vi "Best Focus.vi"(7 "Use Strength?":bool, 8 "error in (no error)":errorcluster, 9 "Inc by":dbl=-0.1 format="%#_13g", 10 "Start":dbl=1.0 format="%#_13g", 11 "Gantry In":refnum<k24>) -> (0 "error out":errorcluster, 2 "max value":dbl, 3 "Gantry Out":refnum<k24>)   [LabVIEW 2021, in "Component Tray.lvclass"]
uses:
  Component Tray.lvclass
  C:/Program Files (x86)/Aerotech/A3200/LabVIEW/2010/Bin/Aerotech.A3200.dll
  Program Files (x86)/Aerotech/A3200/LabVIEW/2010/Bin/Aerotech.A3200.dll
  Controller/Motion/A3200/A3200.lvclass
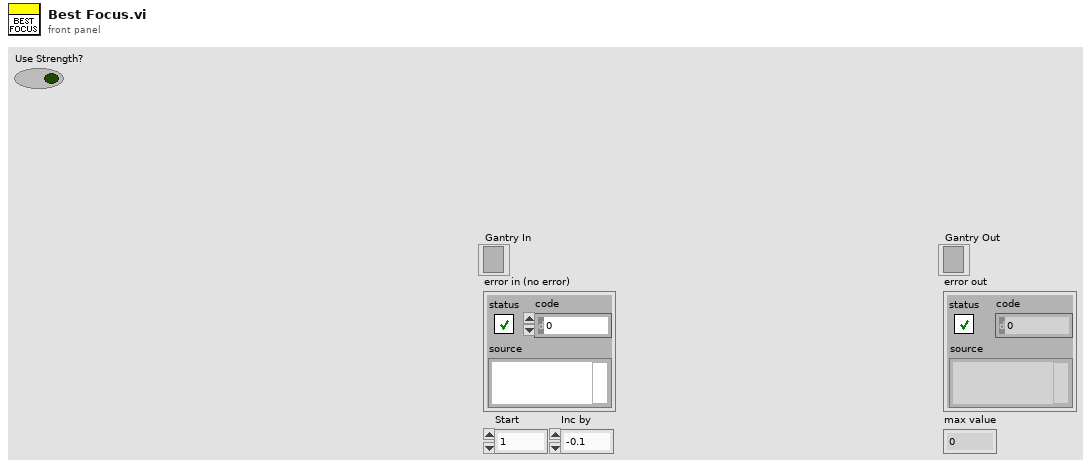
[diagram p1: front panel]
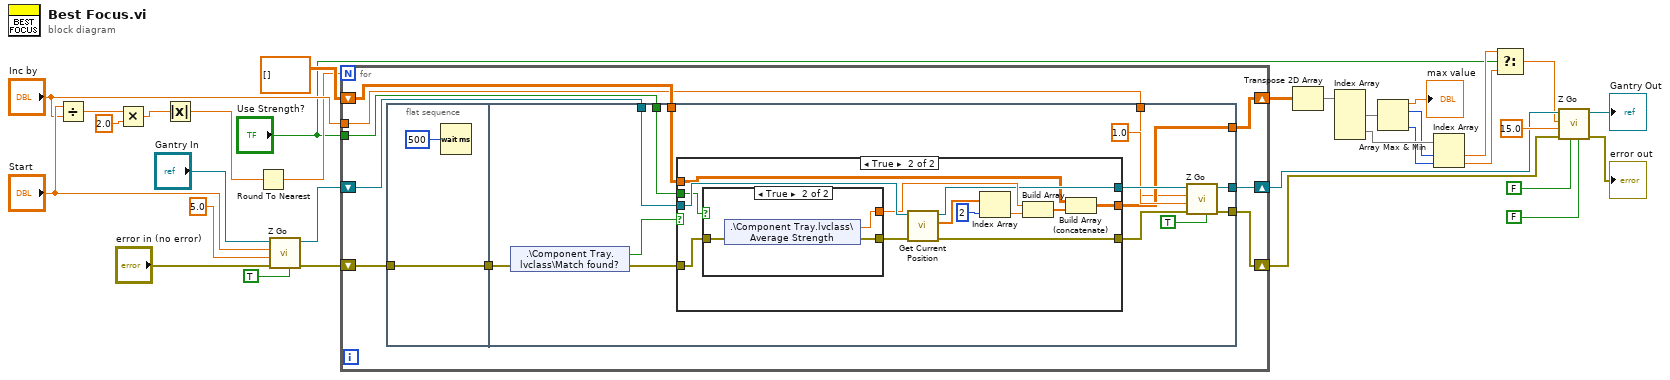
[diagram p0: block diagram]
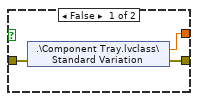
[diagram p3: hidden frame]
diagram:
  n1 = Divide(x="Start", y="Inc by") -> (x/y=w10:dbl)
  n2 = Multiply(x=w10, y=2.0) -> (x*y=w7:dbl)
  n3 = Absolute Value(x=w7) -> (abs(x)=w6:dbl)
  n4 = Round To Nearest(number=w6) -> (nearest integer value=w8:dbl)
  n5 = call "Z Go.vi"("Increment"=TRUE, "error in (no error)"="error in (no error)", "Speed In"=5.0, "Position In"="Start", "Gantry In"="Gantry In") -> ("error out"=w30:errorcluster, "Gantry Out"=w29:refnum<k24>)  [unwired: 3 in, 2 out]
  n6 = for {
    N: w8 -> [_]
    shift-right: [w37] -> w20
    shift-left: w30 -> [w41]
    shift-right: [w38] -> w21
    shift-left: w29 -> [w39]
    shift-right: [w36] -> w19
    shift-left: dbl[][] [] -> [w35]
    tunnel: "Inc by" -> [w34]
    tunnel: "Use Strength?" -> [w33]
    n7 = flat-sequence {
      tunnel: w41 -> [w43]
      tunnel: [w43] -> w40
      tunnel: w39 -> [w55]
      tunnel: w40 -> [w56]
      tunnel: [w51] -> w38
      tunnel: [w50] -> w37
      tunnel: [w47] -> w36
      tunnel: w35 -> [w46]
      tunnel: w34 -> [w45]
      tunnel: w33 -> [w44]
      frame #0 {
        n8 = Wait (ms)(milliseconds to wait=u32 500) -> ()  [unwired: 1 out]
      }
      frame #1 {
        n9 = shared-variable ".\\Component Tray.lvclass\\Match found?"(error in=w56) -> (w57:bool, error out=w54:errorcluster)
        n10 = case shown="True" w57 {
          tunnel: w55 -> [w60 w73]
          tunnel: w54 -> [w59 w71]
          tunnel: [w60 w66] -> w53
          tunnel: [w59 w65] -> w52
          tunnel: [w58 w63] -> w47
          tunnel: w46 -> [w58 w62]
          tunnel: w44 -> [_ w61]
          frame False {
          }
          frame True {
            n11 = case shown="True" w61 {
              tunnel: [w75 w79] -> w72
              tunnel: w71 -> [w76 w78]
              tunnel: [w74 w77] -> w67
              frame False {
                n12 = shared-variable ".\\Component Tray.lvclass\\Standard Variation"(error in=w76) -> (w74:sgl, error out=w75:errorcluster)
              }
              frame True {
                n13 = shared-variable ".\\Component Tray.lvclass\\Average Strength"(error in=w78) -> (w77:dbl, error out=w79:errorcluster)
              }
            }
            n14 = call "Get Current Position.vi"("error in (no error)"=w72, "Gantry In"=w73) -> ("error out"=w65:errorcluster, "XYZTheta Out"=w70:dbl[], "Gantry Out"=w66:refnum<k24>)  [unwired: 7 in]
            n15 = Index Array(array=w70, index=2) -> (element=w68:dbl)
            n16 = Build Array(w67, w68) -> (w64:dbl[])
            n17 = Build Array (concatenate)(w62, w64) -> (w63:dbl[][])
          }
        }
        n18 = call "Z Go.vi"("Increment"=TRUE, "error in (no error)"=w52, "Speed In"=1.0, "Position In"=w45, "Gantry In"=w53) -> ("error out"=w50:errorcluster, "Gantry Out"=w51:refnum<k24>)  [unwired: 3 in, 2 out]
      }
    }
  }
  n19 = Transpose 2D Array(2D array=w19) -> (transposed array=w25:dbl[][])
  n20 = Index Array(array=w25) -> (element #1=w22:dbl[], element #2=w24:dbl[])  [unwired: 4 in]
  n21 = Array Max & Min(array=w22) -> (max value=→"max value":dbl, max index (indices)=w23:i32, min index (indices)=w5:i32)  [unwired: 1 out]
  n22 = Index Array(array=w24, index #1=w23, index #2=w5) -> (element #1=w4:dbl, element #2=w3:dbl)
  n23 = Select(t=w4, s="Use Strength?", f=w3) -> (s? t:f=w2:dbl)
  n24 = call "Z Go.vi"("Increment"=FALSE, "Return Immediately"=FALSE ("Increment"), "error in (no error)"=w20, "Speed In"=15.0 ("Speed"), "Position In"=w2, "Gantry In"=w21) -> ("error out"=→"error out":errorcluster, "Gantry Out"=→"Gantry Out":refnum<k24>)  [unwired: 2 in, 2 out]
